vi "DAQLoop.vi"() -> ()   [LabVIEW 2014]
uses:
  Controls/FHandlerClusterTypedef.ctl
  Controls/FHandlerEnumTypedef.ctl
  Controls/FGVisfileopen.ctl
  Controls/MasterClusterTypedef.ctl
  Controls/MasterEnumTypedef.ctl
  Controls/DataPack.ctl
  Controls/CMWQCluster.ctl
  Controls/CMWQEnum.ctl
panel:
  out "PLC cluster":T1
  out "error out":errorcluster
  in  "error in":errorcluster
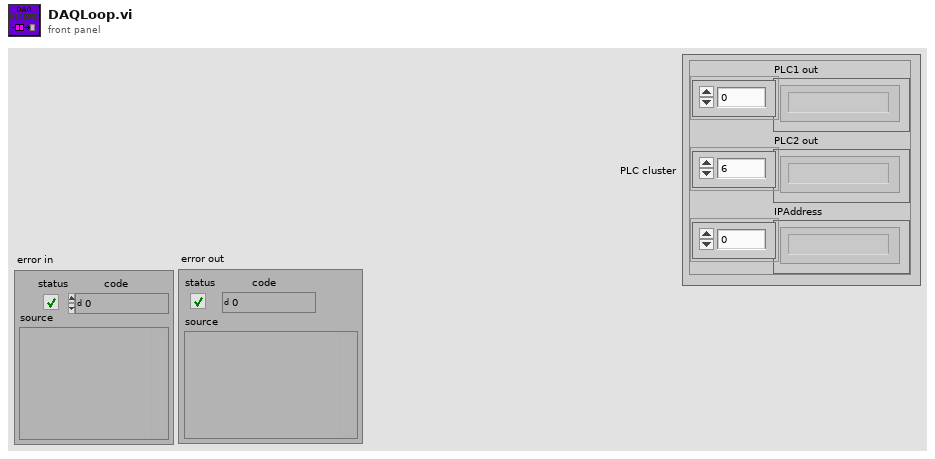
[diagram p1: front panel]
types:
  T1 = cluster{"PLC1 out":string[], "PLC2 out ":string[], "IPAddress":string[]}
  T2 = typedef "DataPack.ctl" = cluster{"DataPack Array":cluster{"Method":string, "PropertyName":string, "Value":string, "Display?":string, "Unit":string}[], "current time":timestamp}
  T3 = typedef "MasterClusterTypedef.ctl" = cluster{"DisplayVariant":variant, "DisplayEnum":T4}
  T4 = typedef "MasterEnumTypedef.ctl" = enum16{"Idle", "Initialize", "StartAcquisition", "StoreAcquisition", "PrintScreen", "AddComment", "ClearTable", "DisplayTable", "DisplayWaveforms", "ExportConfig", "LoadConfig", "Exit"}
  T5 = typedef "FGVisfileopen.ctl" = enum16{"Read", "Write"}
  T6 = typedef "FHandlerClusterTypedef.ctl" = cluster{"File Variant":variant, "FileHandler Enum":T7}
  T7 = typedef "FHandlerEnumTypedef.ctl" = enum16{"InitLog", "CommentLog", "WriteExperimental", "WriteRGA", "WriteAccelerator", "WriteInstrument", "ClearLog", "ReadConfig", "WriteConfig", "ExitFH"}
  T8 = typedef "CMWQCluster.ctl" = cluster{"Variant":variant, "Enum":T9}
  T9 = typedef "CMWQEnum.ctl" = enum16{"Initialise", "Acquire", "Stop"}
  T10 = cluster{"Method":string, "PropertyName":string, "Value":string, "Display?":string, "Unit":string}
  T11 = cluster{"Method":string, "PropertyName":string, "Value":string, "Display?":string, "Unit":string}[]
  T12 = cluster{"Method":string, "Property":string, "URL/IPAddress":string, "Data type":string, "Display?":string, "Unit":string}[]
  T13 = cluster{"231":string[], "225":string[], "IPAddress":string[]}
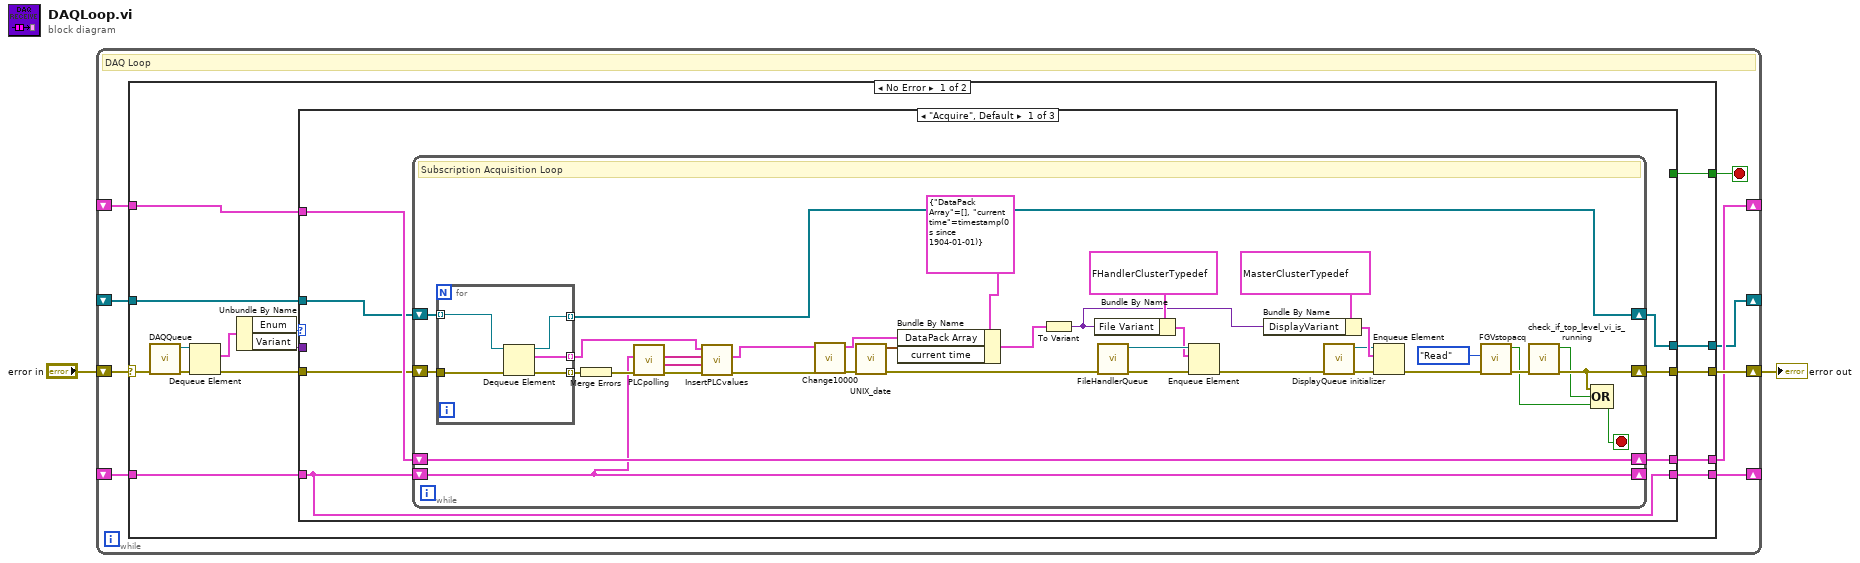
[diagram p0: block diagram]
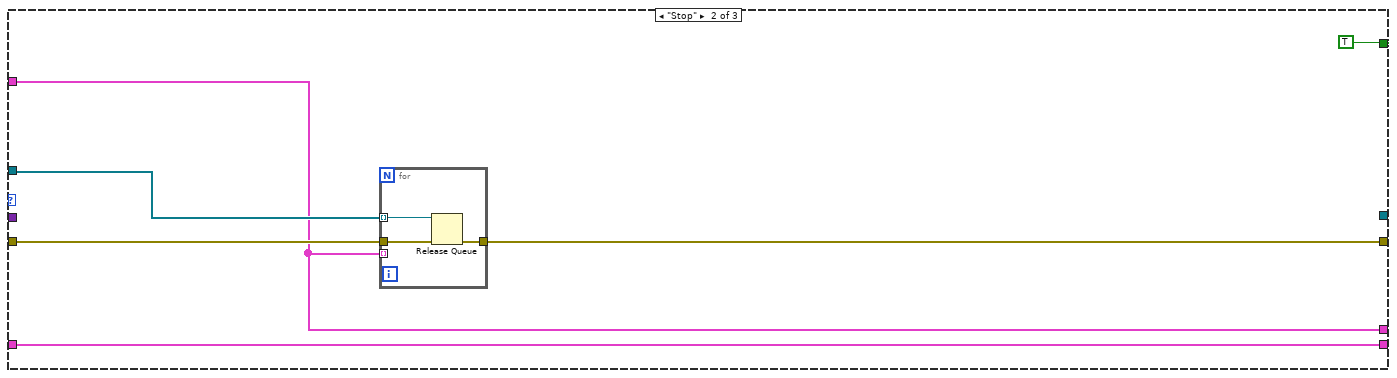
[diagram p2: hidden frame]
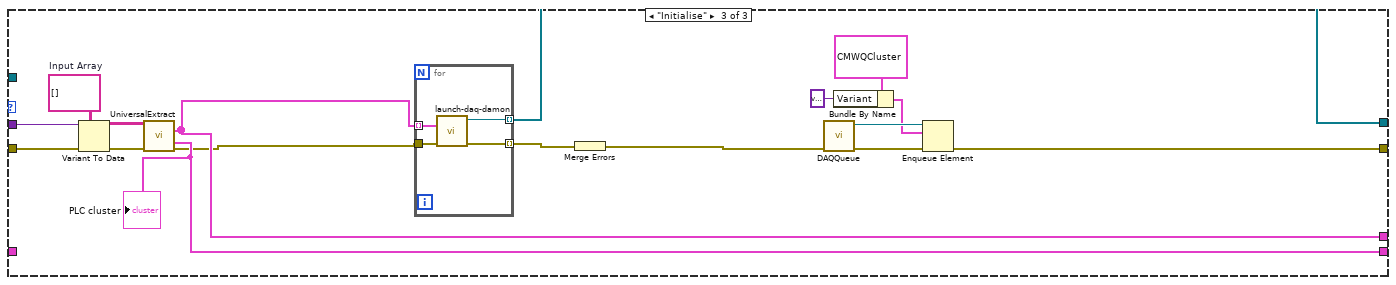
[diagram p3: hidden frame]
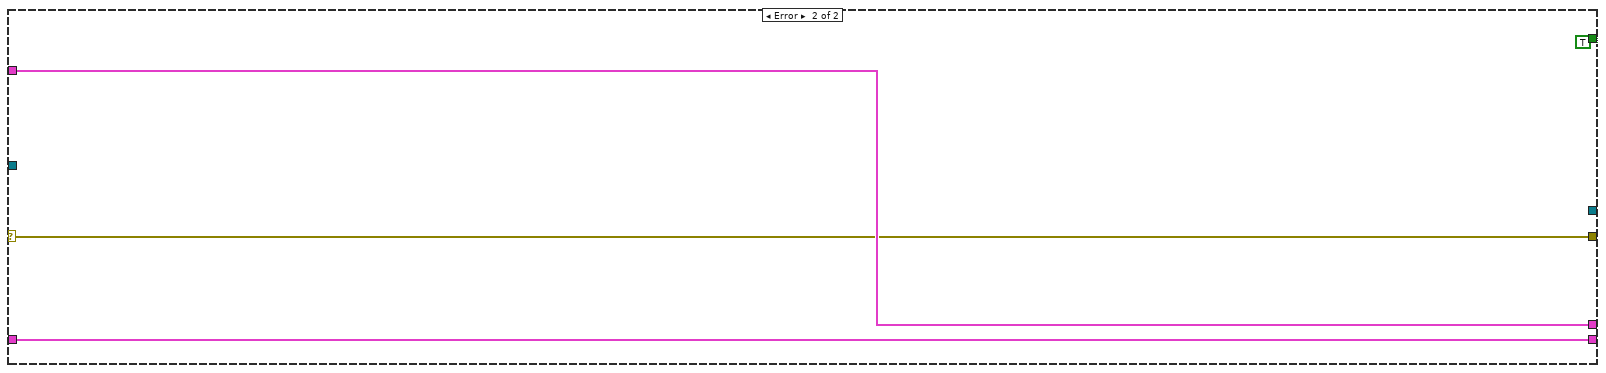
[diagram p4: hidden frame]
diagram:
  n1 = while {
    shift-right: [w10] -> w1
    shift-left: "error in" -> [w11]
    shift-right: [w9] -> _
    shift-left: _ -> [w8]
    shift-right: [w6] -> _
    shift-left: _ -> [w5]
    shift-right: [w4] -> _
    shift-left: _ -> [w3]
    stop <- w7 stop-if-true
    # "DAQ Loop"
    n2 = case shown="No Error" w11 {
      selector: w11 -> [w25 w105]
      tunnel: [w26 w105] -> w10
      tunnel: [w21 w106] -> w9
      tunnel: w8 -> [w20 w106]
      tunnel: [w14 TRUE] -> w7
      tunnel: [w16 _] -> w6
      tunnel: w5 -> [w15 _]
      tunnel: [w13 w104] -> w4
      tunnel: w3 -> [w12 w104]
      frame No Error {
        n3 = call "DAQQueue.vi"("error in"=w25) -> ("error out"=w24:errorcluster, "queue out"=w23:refnum<queue>)  [unwired: 8 in]
        n4 = Dequeue Element(queue=w23, error in (no error)=w24) -> (element=w22:T8, error out=w19:errorcluster)  [unwired: 1 in, 2 out]
        n5 = Unbundle By Name(w22) -> ("Enum"=w17:T9, "Variant"=w18:variant)
        n6 = case shown="\"Acquire\", Default" w17 {
          tunnel: w19 -> [w27 w77 w97]
          tunnel: [w33 w78 w90] -> w26
          tunnel: [w30 w75 w87] -> w21
          tunnel: [_ TRUE _] -> w14
          tunnel: w20 -> [w31 w75 _]
          tunnel: w18 -> [_ _ w96]
          tunnel: [w32 _ w83] -> w16
          tunnel: w15 -> [w28 w76 _]
          tunnel: [w29 w74 w88] -> w13
          tunnel: w12 -> [w29 w74 _]
          frame "Acquire", Default {
            n7 = while {
              shift-right: [w53] -> w33
              shift-left: w27 -> [w43]
              shift-right: [w49] -> w30
              shift-left: w31 -> [w49]
              shift-right: [w39] -> _
              shift-left: w29 -> [w39]
              shift-right: [w55] -> w32
              shift-left: w28 -> [w56]
              stop <- w50 stop-if-true
              # "Subscription Acquisition Loop"
              n8 = for {
                tunnel: w43 -> [w72]
                tunnel: [w69] -> w42 mode=indexing
                tunnel: [w70] -> w36 mode=indexing
                tunnel: w56 -> [w73] mode=indexing
                tunnel: [w71] -> w55 mode=indexing
                n9 = Dequeue Element(queue=w73, error in (no error)=w72) -> (queue out=w71:refnum<queue>, element=w70:T10, error out=w69:errorcluster)  [unwired: 1 in, 1 out]
              }
              n10 = Merge Errors(w42) -> (w41:errorcluster)
              n11 = call "PLCpolling.vi"("error in"=w41, "PLC cluster"=w39) -> ("error out"=w40:errorcluster, "172.18.214.225"=w37:string[], "172.18.214.231"=w38:string[])  [unwired: 7 in]
              n12 = call "InsertPLCvalues.vi"("172.18.214.225"=w37, "172.18.214.231"=w38, "Array"=w36) -> ("OutputValues"=w34:T11)  [unwired: 8 in]
              n13 = call "Change10000.vi"("error in"=w40, "Input"=w34) -> ("error out"=w44:errorcluster, "Output data array"=w35:T11)  [unwired: 8 in]
              n14 = call "UNIX_date.vi"("error in (no error)"=w44) -> ("error out"=w62:errorcluster, "current time"=w58:timestamp)  [unwired: 9 in]
              n15 = Bundle By Name(cluster=T2 {"DataPack Array"=[], "current time"=timestamp(0 s since 1904-01-01)}, "DataPack Array"=w35, "current time"=w58) -> (w57:T2)
              n16 = To Variant(anything=w57) -> (Variant=w54:variant)
              n17 = Bundle By Name(cluster=T6 {"File Variant"=variant, "FileHandler Enum"=enum."WriteExperimental"} ("element"), "File Variant"=w54) -> (w65:T6)
              n18 = call "FileHandlerQueue.vi"("error in"=w62) -> ("error out"=w67:errorcluster, "queue out"=w68:refnum<queue>)  [unwired: 8 in]
              n19 = Enqueue Element(queue=w68, element=w65, error in (no error)=w67) -> (error out=w45:errorcluster)  [unwired: 1 in, 2 out]
              n20 = Bundle By Name(cluster=T3 {"DisplayVariant"=variant, "DisplayEnum"=enum."DisplayWaveforms"} ("element"), "DisplayVariant"=w54) -> (w59:T3)
              n21 = call "DisplayQueue initializer.vi"("error in"=w45) -> ("error out"=w46:errorcluster, "queue out"=w47:refnum<queue>)  [unwired: 8 in]
              n22 = Enqueue Element(queue=w47, element=w59, error in (no error)=w46) -> (error out=w61:errorcluster)  [unwired: 1 in, 2 out]
              n23 = call "FGVstopacq.vi"("error in"=w61, "Write from FGV or Read from FGV?"=FGVisfileopen."Read") -> ("error out"=w64:errorcluster, "Output Value"=w51:bool)  [unwired: 8 in]
              n24 = call "check_if_top_level_vi_is_running.vi"("error in (no error)"=w64) -> ("error out"=w53:errorcluster, "stop?"=w52:bool)  [unwired: 9 in]
              n25 = Compound Arithmetic op=OR(w53, w52, w51) -> (w50:bool)
            }
          }
          frame "Stop" {
            n26 = for {
              tunnel: w77 -> [w80]
              tunnel: [w81] -> w78
              tunnel: w75 -> [_] mode=indexing
              tunnel: w76 -> [w82] mode=indexing
              n27 = Release Queue(queue=w82, error in (no error)=w80) -> (error out=w81:errorcluster)  [unwired: 1 in, 2 out]
            }
          }
          frame "Initialise" {
            w95 = string[][] []  # Input Array
            n28 = Variant To Data(error in=w97, type=w95, Variant=w96) -> (data=w93:string[][], error out=w94:errorcluster)
            n29 = call "UniversalExtract.vi"("Input Array"=w93, "Error In"=w94) -> ("Data Parameters"=w87:T12, "PLC cluster"=w88:T13, "Error Out"=w86:errorcluster)  [unwired: 11 in]
            "PLC cluster" <- w88
            n30 = for {
              tunnel: w86 -> [w103]
              tunnel: [w101] -> w84 mode=indexing
              tunnel: w87 -> [w100] mode=indexing
              tunnel: [w102] -> w83 mode=indexing
              n31 = call "launch-daq-damon.vi"("error in (no error)"=w103, "Parameters"=w100) -> ("error out"=w101:errorcluster, "queue out"=w102:refnum<queue>)  [unwired: 8 in]
            }
            n32 = Merge Errors(w84) -> (w85:errorcluster)
            n33 = call "DAQQueue.vi"("error in"=w85) -> ("error out"=w99:errorcluster, "queue out"=w98:refnum<queue>)  [unwired: 8 in]
            n34 = Bundle By Name(cluster=T8 {"Variant"=variant, "Enum"=enum."Acquire"}, "Variant"=variant) -> (w91:T8)
            n35 = Enqueue Element(queue=w98, element=w91, error in (no error)=w99) -> (error out=w90:errorcluster)  [unwired: 1 in, 2 out]
          }
        }
      }
      frame Error {
      }
    }
  }
  "error out" <- w1
